vi "StringifiedData.vi"(8 "error in (no error)":errorcluster, 11 "I32ArrayMsg in":refnum<class "I32ArrayMsg.lvclass">) -> (0 "error out":errorcluster, 2 "Stringified Data":string, 3 "I32ArrayMsg out":refnum<class "I32ArrayMsg.lvclass">)   [LabVIEW 2018, in "LapDog.Messaging.v3.NativeArrays.lvlib" / "I32ArrayMsg.lvclass"]
doc: "This VI is used for the message probe. Child classes may override it and provide the message data in string format or a short string describing the data the message contains. This string will be displayed in the probe window."
uses:
  I32ArrayMsg.lvclass
  I32ArrayMsg.lvclass/I32ArrayMsg.ctl
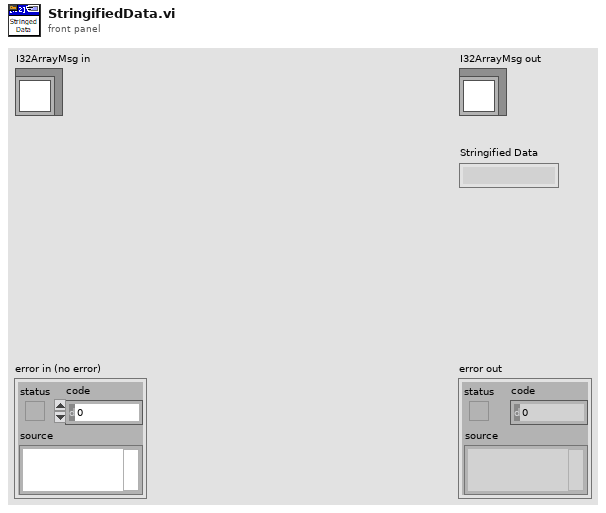
[diagram p1: front panel]
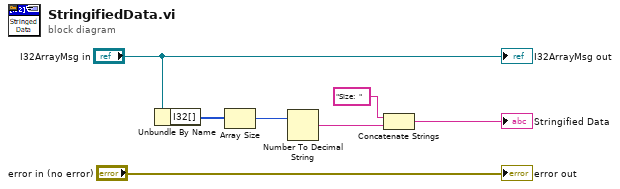
[diagram p0: block diagram]
diagram:
  n1 = Unbundle By Name("I32ArrayMsg in") -> ("I32[]"=w6:i32[])
  n2 = Array Size(array=w6) -> (size(s)=w5:i32)
  n3 = Number To Decimal String(number=w5) -> (decimal integer string=w3:string)  [unwired: 1 in]
  n4 = Concatenate Strings("Size:  " ("string"), w3) -> (→"Stringified Data":string)
  "error out" <- "error in (no error)"
  "I32ArrayMsg out" <- "I32ArrayMsg in"
